vi "GenerateMsgClassFilename.vi"(11 "Target Method":string) -> (3 "Msg Class File Name":string)   [LabVIEW 2016, in "CS++Actor.lvlib" / "CS++Actor.lvclass"]
doc: "Small helper Vi to generate the new Msg file name."
uses:
  CS++Actor.lvclass
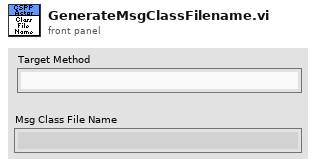
[diagram p1: front panel]
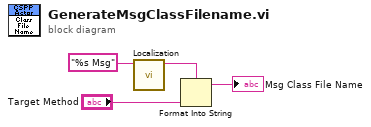
[diagram p0: block diagram]
diagram:
  n1 = call "Localization.vi"("Unlocalized"="%s Msg" ("Name of new Message Class (without .lvclass file extension)")) -> ("Localized"=w1:string)  [unwired: 10 in]
  n2 = Format Into String(format string=w1, "Target Method") -> (resulting string=→"Msg Class File Name":string)  [unwired: 2 in, 1 out]
